vi "Read Helper Stop Notifier.vi"(8 "error in (no error)":errorcluster, 11 "Process In":refnum<class "Process.lvclass">) -> (0 "error out":errorcluster, 2 "Helper Stop Notifier":refnum<notifier>, 3 "Process Out":refnum<class "Process.lvclass">)   [LabVIEW 2020, in "Process.lvclass"]
doc: "This method reads the helper loop stop notifier used by the helper loop interface. This method is a framework method and not meant to be used for other purposes."
uses:
  Process.lvclass
  Process.lvclass/Process.ctl
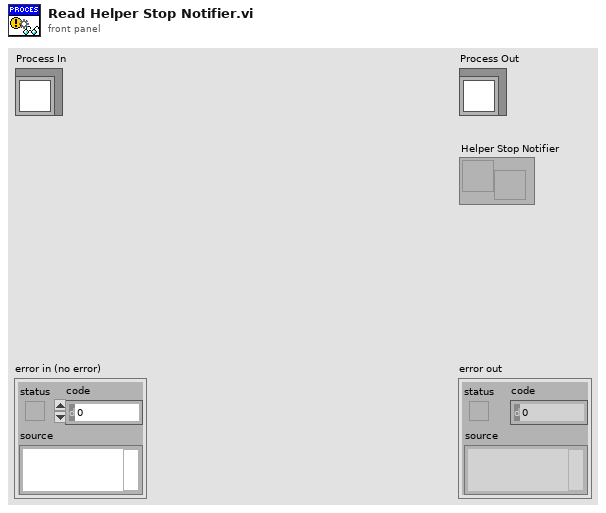
[diagram p1: front panel]
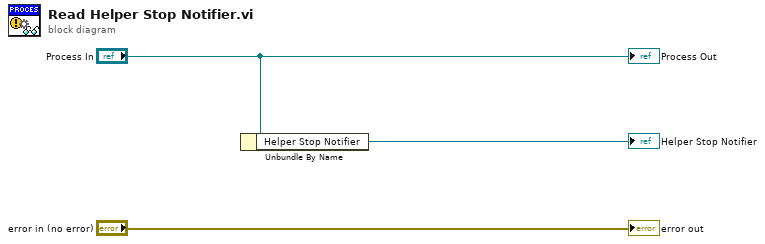
[diagram p0: block diagram]
diagram:
  n1 = Unbundle By Name("Process In") -> ("Helper Stop Notifier"=→"Helper Stop Notifier":refnum<notifier>)
  "error out" <- "error in (no error)"
  "Process Out" <- "Process In"
